vi "DataVIS_Decimate+Fill_Intensity_Plot.vi"(7 "Voffset -2T":dbl, 8 "error in (no error)":errorcluster, 9 "fake point value":dbl, 10 "Decimate Controls":T1, 11 "X and Y Arrays to decimate":T2(array[cluster])) -> (0 "error out":errorcluster, 1 "Offset X Low":dbl, 2 "Decimated X values":dbl[](array[numeric]), 3 "Arr of Y arrays (intensity info)":dbl[][](array[numeric]))   [LabVIEW 2016]
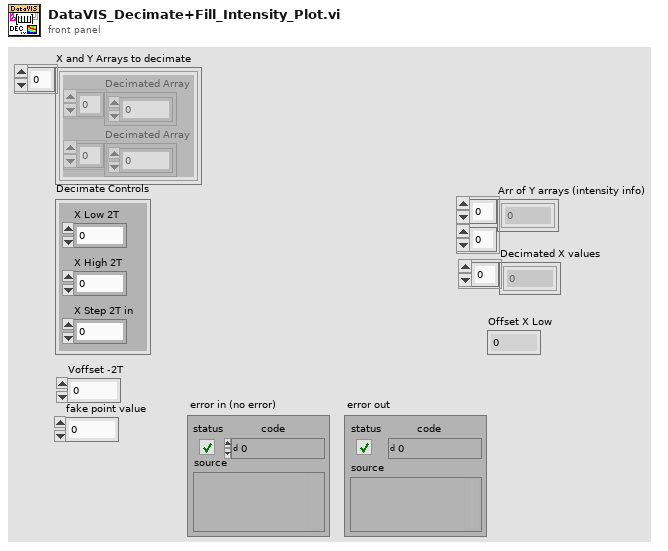
[diagram p1: front panel]
types:
  T1 = cluster{"X Low 2T":dbl, "X High 2T":dbl, "X Step 2T in":dbl}
  T2 = cluster{"Decimated Array":dbl[], "Decimated Array":dbl[]}[]
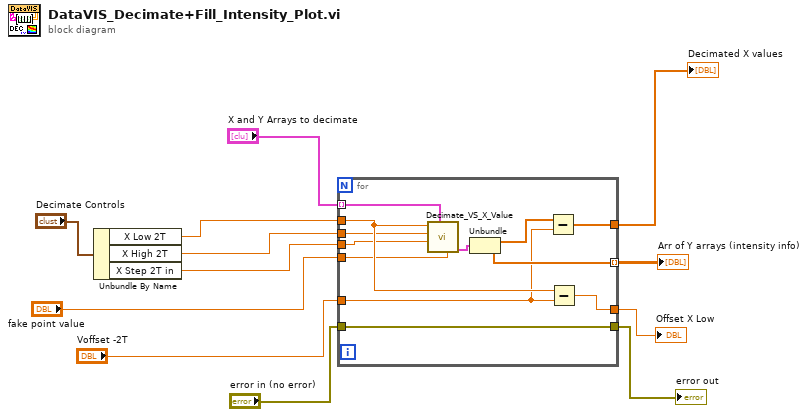
[diagram p0: block diagram]
diagram:
  n1 = Unbundle By Name("Decimate Controls") -> ("X Low 2T"=w5:dbl, "X High 2T"=w4:dbl, "X Step 2T in"=w3:dbl)
  n2 = for {
    tunnel: [w22] -> w7
    tunnel: [w23] -> w10
    tunnel: "X and Y Arrays to decimate" -> [w17] mode=indexing
    tunnel: [w21] -> w9 mode=indexing
    tunnel: w5 -> [w20]
    tunnel: w4 -> [w19]
    tunnel: w3 -> [w18]
    tunnel: "Voffset -2T" -> [w15]
    tunnel: "fake point value" -> [w14]
    tunnel: "error in (no error)" -> [w13]
    tunnel: [w13] -> w1
    n3 = call <userlib>:"Decimate_VS_X_Value.vi"("fake point value"=w14, "XY Graph kind 1"=w17, "X Step"=w18, "X High"=w19, "X Low"=w20) -> ("Interpolated"=w16:cluster{dbl[], dbl[]})  [unwired: 5 in, 1 out]
    n4 = Unbundle(w16) -> (w24:dbl[], w21:dbl[])
    n5 = Subtract(x=w24, y=w15) -> (x-y=w23:dbl[])
    n6 = Subtract(x=w20, y=w15) -> (x-y=w22:dbl)
  }
  "Decimated X values" <- w10
  "Arr of Y arrays (intensity info)" <- w9
  "Offset X Low" <- w7
  "error out" <- w1
